vi "CompressAndUpdate(Path).vi"(7 "force CVT update (false)":bool, 8 "error in":errorcluster, 10 "Path":path, 11 "command or variable name":string) -> (0 "error out":errorcluster)   [LabVIEW 2011]
panel:
  out "string":string
  in  "precision (6)":i16
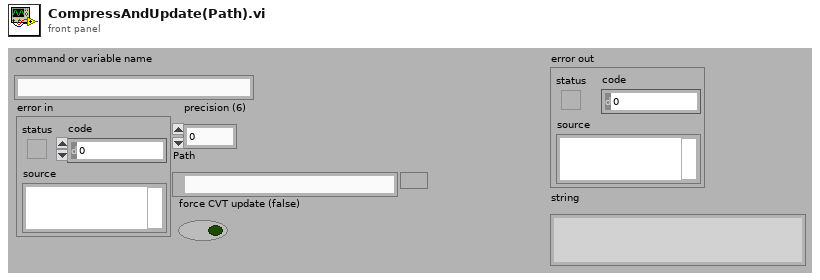
[diagram p1: front panel]
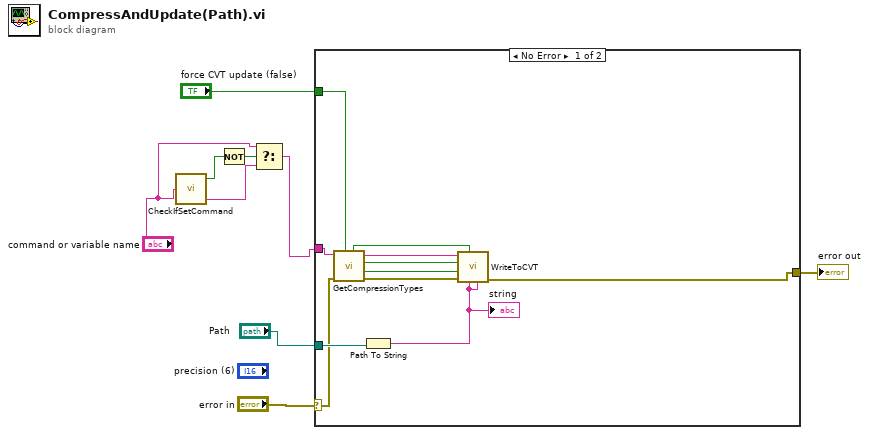
[diagram p0: block diagram]
diagram:
  n1 = call "CheckIfSetCommand.vi"("Command"="command or variable name") -> ("setCommand?"=w5:bool, "variable"=w4:string)  [unwired: 1 out]
  n2 = Not(x=w5) -> (.not. x?=w6:bool)
  n3 = Select(t="command or variable name", s=w6, f=w4) -> (s? t:f=w2:string)
  n4 = case shown="No Error" "error in" {
    selector: "error in" -> [w18 w21]
    tunnel: [w10 w21] -> w9
    tunnel: w2 -> [w20 _]
    tunnel: "Path" -> [w19 _]
    tunnel: "force CVT update (false)" -> [w11 _]
    frame No Error {
      n5 = call "GetCompressionTypes.vi"("force CVT update"=w11, "error in"=w18, "variable"=w20) -> ("error out"=w14:errorcluster, "non compressed"=w15:bool, "compressed"=w16:bool, "variable out"=w17:string, "force CVT update out"=w12:bool)  [unwired: 4 in]
      n6 = Path To String(path=w19) -> (string=w13:string)
      "string" <- w13
      n7 = call "WriteToCVT.vi"("non compressed string"=w13, "compressed string"=w13, "force CVT update"=w12, "error in"=w14, "non compressed"=w15, "compressed"=w16, "variable"=w17) -> ("error out"=w10:errorcluster)  [unwired: 4 in]
    }
    frame Error {
    }
  }
  "error out" <- w9
